vi "ATF-Pump-Index getter Analog.vi"(9 "output cluster":T1, 10 "AI Y  data":dbl[](array[numeric]), 11 "AI Channels Name":string[](array[string])) -> (3 "Analog data":dbl)   [LabVIEW 2022 SP3]
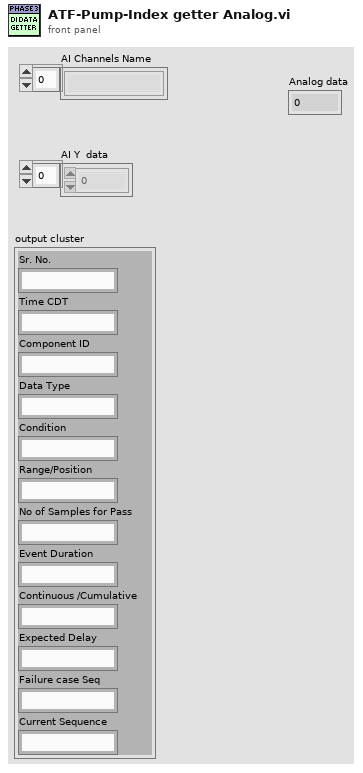
[diagram p1: front panel]
types:
  T1 = cluster{"Sr. No.":string, "Time CDT":string, "Component ID":string, "Data Type":string, "Condition":string, "Range/Position":string, "No of Samples for Pass":string, "Event Duration":string, "Continuous /Cumulative":string, "Expected Delay":string, "Failure case Seq":string, "Current Sequence":string}
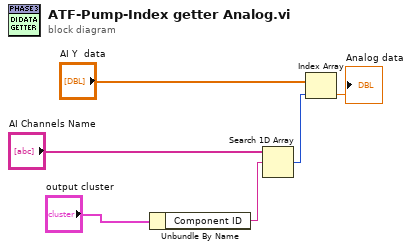
[diagram p0: block diagram]
diagram:
  n1 = Unbundle By Name("output cluster") -> ("Component ID"=w3:string)
  n2 = Search 1D Array(1D array="AI Channels Name", element=w3) -> (index of element=w2:i32)  [unwired: 1 in]
  n3 = Index Array(array="AI Y  data", index=w2) -> (element=→"Analog data":dbl)
